vi "Data Polar Vectors.vi"(8 "error in (no error)":errorcluster, 10 "VI_Polar_array":sgl[](array[numeric]), 11 "Polar_VI":T1) -> (0 "error out":errorcluster, 2 "current vectors":cdb[](array[numeric]), 3 "voltage vectors":cdb[](array[numeric]))   [LabVIEW 2018]
uses:
  Controls/Polar_cluster.ctl
  <vilib>/addons/Electrical Power/Basic/NI_EP_Basic.lvlib
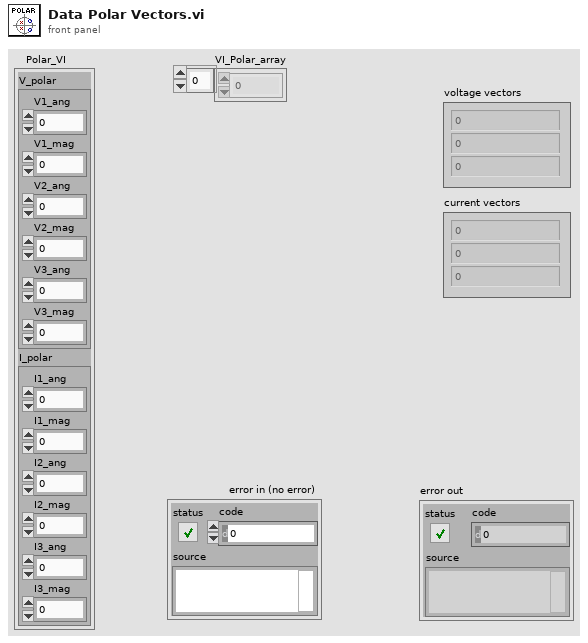
[diagram p1: front panel]
types:
  T1 = typedef "Polar_cluster.ctl" = cluster{"V_polar":cluster{"V1_ang":sgl, "V1_mag":sgl, "V2_ang":sgl, "V2_mag":sgl, "V3_ang":sgl, "V3_mag":sgl}, "I_polar":cluster{"I1_ang":sgl, "I1_mag":sgl, "I2_ang":sgl, "I2_mag":sgl, "I3_ang":sgl, "I3_mag":sgl}}
  T2 = cluster{"V1_ang":sgl, "V1_mag":sgl, "V2_ang":sgl, "V2_mag":sgl, "V3_ang":sgl, "V3_mag":sgl}
  T3 = cluster{"I1_ang":sgl, "I1_mag":sgl, "I2_ang":sgl, "I2_mag":sgl, "I3_ang":sgl, "I3_mag":sgl}
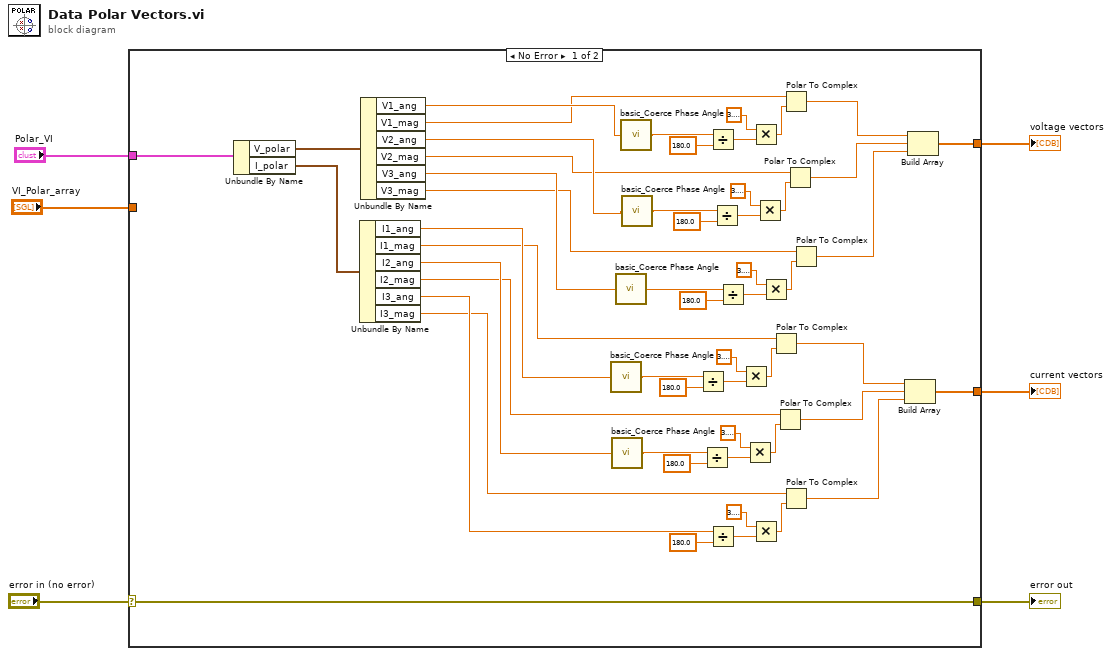
[diagram p0: block diagram]
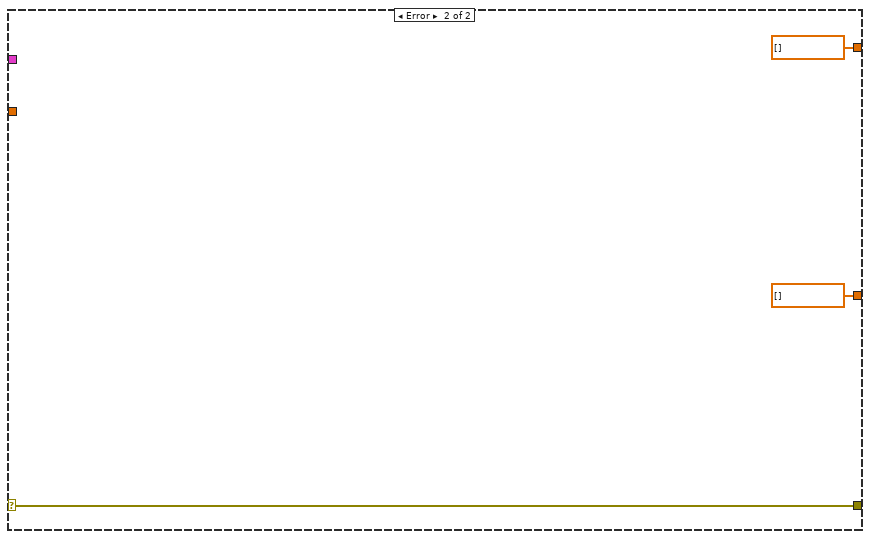
[diagram p2: hidden frame]
diagram:
  n1 = case shown="No Error" "error in (no error)" {
    selector: "error in (no error)" -> [w9 w62]
    tunnel: [w44 cdb[] []] -> w6
    tunnel: [w23 cdb[] []] -> w5
    tunnel: "Polar_VI" -> [w22 _]
    tunnel: [w9 w62] -> w3
    tunnel: "VI_Polar_array" -> [_ _]
    frame No Error {
      n2 = Unbundle By Name(w22) -> ("V_polar"=w8:T2, "I_polar"=w7:T3)
      n3 = Unbundle By Name(w7) -> ("I1_ang"=w17:sgl, "I1_mag"=w16:sgl, "I2_ang"=w15:sgl, "I2_mag"=w14:sgl, "I3_ang"=w13:sgl, "I3_mag"=w12:sgl)
      n4 = Unbundle By Name(w8) -> ("V1_ang"=w21:sgl, "V1_mag"=w20:sgl, "V2_ang"=w19:sgl, "V2_mag"=w18:sgl, "V3_ang"=w11:sgl, "V3_mag"=w10:sgl)
      n5 = call <vilib>:"basic_Coerce Phase Angle.vi"("Phase Angle"=w17) -> ("Phase Angle (-180 to 180)"=w39:dbl)  [unwired: 4 in]
      n6 = call <vilib>:"basic_Coerce Phase Angle.vi"("Phase Angle"=w15) -> ("Phase Angle (-180 to 180)"=w40:dbl)  [unwired: 4 in]
      n7 = call <vilib>:"basic_Coerce Phase Angle.vi"("Phase Angle"=w11) -> ("Phase Angle (-180 to 180)"=w41:dbl)  [unwired: 4 in]
      n8 = call <vilib>:"basic_Coerce Phase Angle.vi"("Phase Angle"=w21) -> ("Phase Angle (-180 to 180)"=w43:dbl)  [unwired: 4 in]
      n9 = call <vilib>:"basic_Coerce Phase Angle.vi"("Phase Angle"=w19) -> ("Phase Angle (-180 to 180)"=w42:dbl)  [unwired: 4 in]
      n10 = Divide(x=w39, y=180.0) -> (x/y=w28:dbl)
      n11 = Divide(x=w40, y=180.0) -> (x/y=w33:dbl)
      n12 = Divide(x=w43, y=180.0) -> (x/y=w58:dbl)
      n13 = Divide(x=w13, y=180.0) -> (x/y=w36:dbl)
      n14 = Divide(x=w42, y=180.0) -> (x/y=w53:dbl)
      n15 = Divide(x=w41, y=180.0) -> (x/y=w50:dbl)
      n16 = Multiply(x=3.141592653589793, y=w28) -> (x*y=w30:dbl)
      n17 = Multiply(x=3.141592653589793, y=w33) -> (x*y=w31:dbl)
      n18 = Multiply(x=3.141592653589793, y=w58) -> (x*y=w56:dbl)
      n19 = Multiply(x=3.141592653589793, y=w36) -> (x*y=w38:dbl)
      n20 = Multiply(x=3.141592653589793, y=w53) -> (x*y=w55:dbl)
      n21 = Multiply(x=3.141592653589793, y=w50) -> (x*y=w48:dbl)
      n22 = Polar To Complex(1:w30, 2:w16) -> (0:w26:cdb)
      n23 = Polar To Complex(1:w31, 2:w14) -> (0:w25:cdb)
      n24 = Polar To Complex(1:w56, 2:w20) -> (0:w47:cdb)
      n25 = Polar To Complex(1:w38, 2:w12) -> (0:w24:cdb)
      n26 = Polar To Complex(1:w55, 2:w18) -> (0:w46:cdb)
      n27 = Polar To Complex(1:w48, 2:w10) -> (0:w45:cdb)
      n28 = Build Array(w26, w25, w24) -> (w23:cdb[])
      n29 = Build Array(w47, w46, w45) -> (w44:cdb[])
    }
    frame Error {
    }
  }
  "voltage vectors" <- w6
  "current vectors" <- w5
  "error out" <- w3
